vi "LaunchLogUI.vi"() -> ()   [LabVIEW 2014, in "zsLaunch.lvlib" / "Launcher.lvclass"]
uses:
  Launcher.lvclass
  EventsLogUI_lib/State Pattern UI/LogUI.lvclass
  <vilib>/ActorFramework/Actor/Actor.lvclass
panel:
  out "error out":errorcluster caption="错误输出"
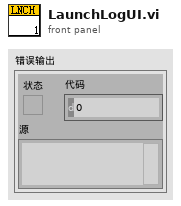
[diagram p1: front panel]
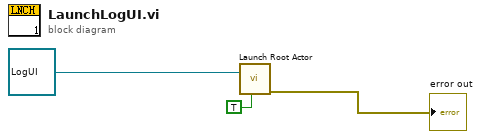
[diagram p0: block diagram]
diagram:
  n1 = call <vilib>:"Launch Root Actor.vi"("Open Actor Core front panel? (F)"=TRUE, "Actor"=refnum<class "LogUI.lvclass"> refnum ("EventsLogUI.lvlib:LogUI.lvclass")) -> ("error out"=→"error out":errorcluster)  [unwired: 8 in, 1 out]
